vi "push array string.vi"(0 "Element":string, 7 "Array":string[](array[string])) -> (8 "Array out":string[](array[string]))   [LabVIEW 2010]
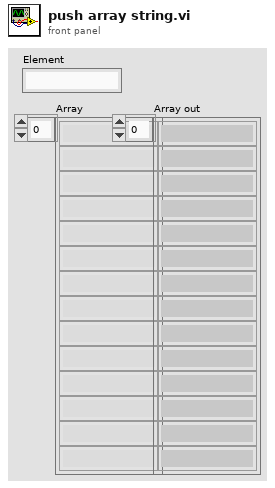
[diagram p1: front panel]
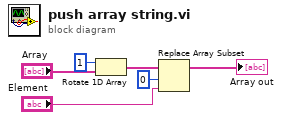
[diagram p0: block diagram]
diagram:
  n1 = Rotate 1D Array(1:"Array", 2:1 ("n")) -> (0:w2:string[])
  n2 = Replace Array Subset(array=w2, new element="Element", index=0 ("Index")) -> (→"Array out":string[])
